vi "Receive NS connection.vi"(8 "error in (no error)":errorcluster, 10 "NS Connection":bool, 11 "Cobra GUI in":refnum<class "Cobra GUI.lvclass">) -> (0 "error out":errorcluster, 3 "Cobra GUI out":refnum<class "Cobra GUI.lvclass">)   [LabVIEW 2019, in "Cobra GUI.lvlib" / "Cobra GUI.lvclass"]
uses:
  Cobra GUI.lvclass
  Network Stream/Network Stream Messages/Read Dataset Msg/Read Dataset Msg.lvclass
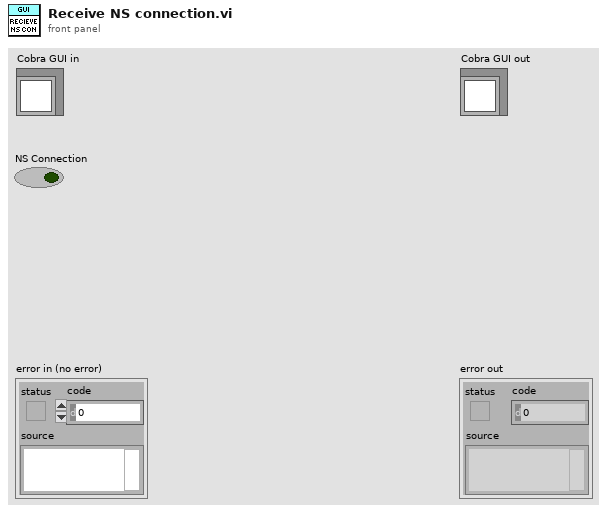
[diagram p1: front panel]
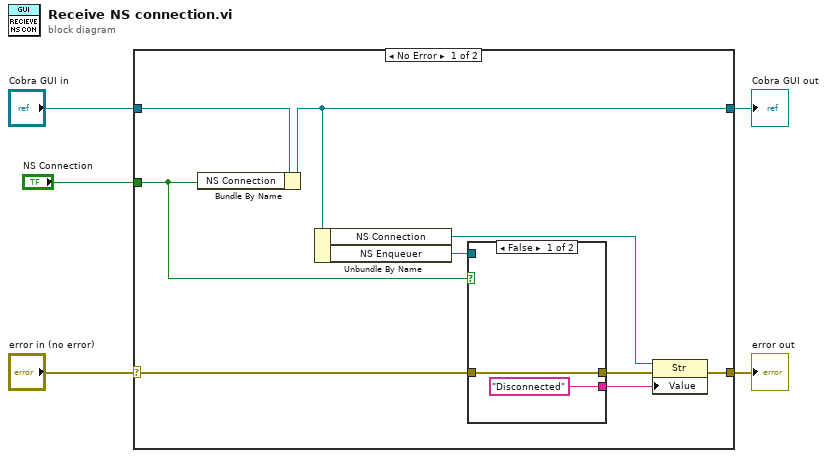
[diagram p0: block diagram]
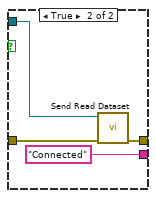
[diagram p2: hidden frame]
diagram:
  n1 = case shown="No Error" "error in (no error)" {
    selector: "error in (no error)" -> [w8 w22]
    tunnel: [w10 w22] -> w4
    tunnel: [w13 w21] -> w2
    tunnel: "Cobra GUI in" -> [w14 w21]
    tunnel: "NS Connection" -> [w12 _]
    frame No Error {
      n2 = Bundle By Name(cluster=w14, "NS Connection"=w12) -> (w13:refnum<class "Cobra GUI.lvclass">)
      n3 = Unbundle By Name(w13) -> ("NS Connection"=w7:refnum<vi>, "NS Enqueuer"=w6:refnum<class "Message Enqueuer.lvclass">)
      n4 = case shown="False" w12 {
        tunnel: ["Disconnected" ("System Info") "Connected" ("System Info")] -> w11
        tunnel: [w15 w19] -> w9
        tunnel: w8 -> [w15 w18]
        tunnel: w6 -> [_ w17]
        frame False {
        }
        frame True {
          n5 = call "Send Read Dataset.vi"("error in (no error)"=w18, "Message Enqueuer"=w17) -> ("error out"=w19:errorcluster)  [unwired: 8 in, 1 out]
        }
      }
      n6 = property class="Str"(reference=w7, error in=w9, "Value"=w11) -> (error out=w10:errorcluster)  [unwired: 1 out]
    }
    frame Error {
    }
  }
  "error out" <- w4
  "Cobra GUI out" <- w2
